vi "TimerVI.vi"(7 "Command":enum16{"GetTime", "Reset"}(ring), 8 "error in (no error)":errorcluster, 10 "Autoreset ?":bool, 11 "Time Target (s)":dbl) -> (0 "error out":errorcluster, 2 "Time has elapsed?":bool, 3 "Elapsed Time":dbl)   [LabVIEW 2017, in "MainFrameLib.lvlib"]
uses:
  MainFrameLib.lvlib
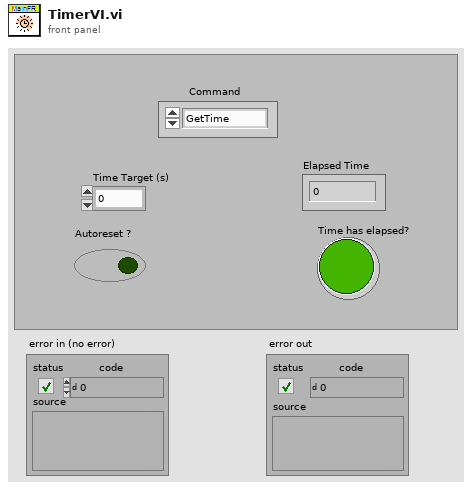
[diagram p1: front panel]
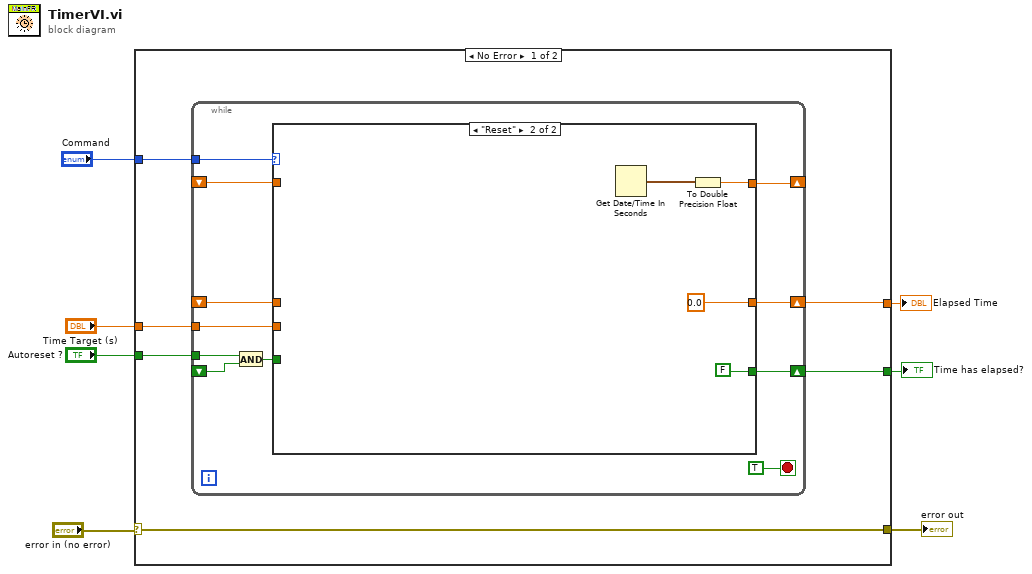
[diagram p0: block diagram]
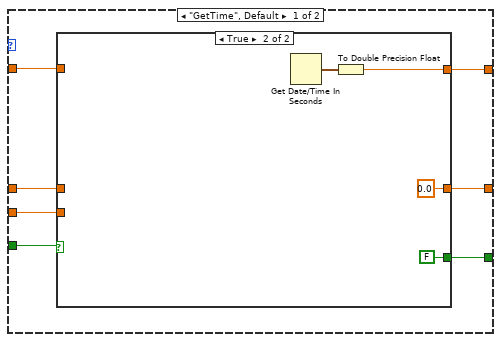
[diagram p2: hidden frame]
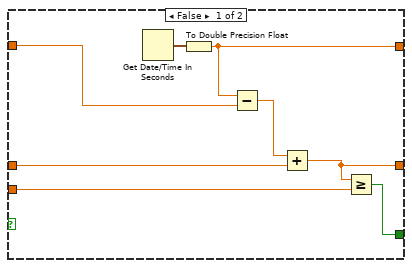
[diagram p3: hidden frame]
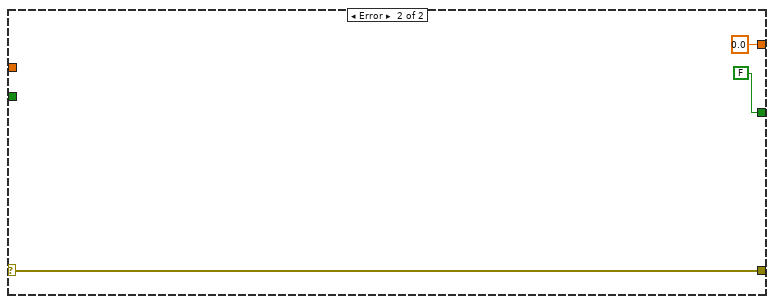
[diagram p4: hidden frame]
diagram:
  n1 = case shown="No Error" "error in (no error)" {
    selector: "error in (no error)" -> [w13 w50]
    tunnel: [w13 w50] -> w6
    tunnel: "Command" -> [w12 _]
    tunnel: "Time Target (s)" -> [w11 _]
    tunnel: [w10 FALSE] -> w3
    tunnel: [w9 0.0] -> w2
    tunnel: "Autoreset ?" -> [w8 _]
    frame No Error {
      n2 = while {
        tunnel: w12 -> [w23]
        tunnel: w11 -> [w22]
        shift-right: [w21] -> _
        shift-left: _ -> [w20]
        shift-right: [w19] -> w9
        shift-left: _ -> [w18]
        shift-right: [w17] -> w10
        shift-left: _ -> [w16]
        tunnel: w8 -> [w15]
        stop <- TRUE stop-if-true
        n3 = And(x=w15, y=w16) -> (x .and. y?=w14:bool)
        n4 = case shown="\"Reset\"" w23 {
          tunnel: w22 -> [w27 _]
          tunnel: [w31 w46] -> w21
          tunnel: w20 -> [w30 _]
          tunnel: [w28 0.0] -> w19
          tunnel: w18 -> [w29 _]
          tunnel: [w26 FALSE] -> w17
          tunnel: w14 -> [w25 _]
          frame "GetTime", Default {
            n5 = case shown="True" w25 {
              tunnel: [w38 w40] -> w31
              tunnel: w30 -> [w37 _]
              tunnel: w29 -> [w35 _]
              tunnel: [w34 0.0] -> w28
              tunnel: w27 -> [w33 _]
              tunnel: [w32 FALSE] -> w26
              frame False {
                n6 = Get Date/Time In Seconds() -> (seconds since 1Jan1904=w39:timestamp)
                n7 = To Double Precision Float(number=w39) -> (double precision float=w38:dbl)
                n8 = Subtract(x=w38, y=w37) -> (x-y=w36:dbl)
                n9 = Add(x=w36, y=w35) -> (x+y=w34:dbl)
                n10 = Greater Or Equal?(x=w34, y=w33) -> (x >= y?=w32:bool)
              }
              frame True {
                n11 = Get Date/Time In Seconds() -> (seconds since 1Jan1904=w41:timestamp)
                n12 = To Double Precision Float(number=w41) -> (double precision float=w40:dbl)
              }
            }
          }
          frame "Reset" {
            n13 = Get Date/Time In Seconds() -> (seconds since 1Jan1904=w47:timestamp)
            n14 = To Double Precision Float(number=w47) -> (double precision float=w46:dbl)
          }
        }
      }
    }
    frame Error {
    }
  }
  "error out" <- w6
  "Time has elapsed?" <- w3
  "Elapsed Time" <- w2
